vi "PlaceChild.vi"(0 "reference in":refnum<class "VGrid.lvclass">, 5 "error in (no error)":errorcluster) -> (14 "reference out":refnum<class "VGrid.lvclass">, 19 "error out":errorcluster)   [LabVIEW 2019, in "VGrid.lvclass"]
uses:
  VGrid.lvclass
  C:/Users/Taylor.Hillegeist/OneDrive - Ultra/LabVIEW/Pgui2/Pgui_Obj_class/Pgui_Obj.lvclass
  Pgui_Obj_class/Pgui_Obj.lvclass
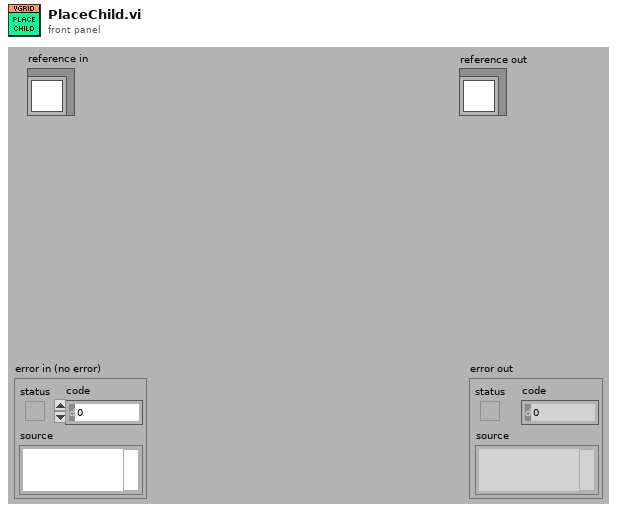
[diagram p1: front panel]
types:
  T1 = cluster{"left":i16, "top":i16, "right":i16, "bottom":i16}
  T2 = typedef "Pgui_Obj.lvclass/ObjectAttributes.ctl" = cluster{"Children":refnum<class "Pgui_Obj.lvclass">[], "Draw Instr":picture, "Params":cluster{"left":i16, "top":i16, "right":i16, "bottom":i16}, "Parent_Pgui_Obj":refnum<class "Pgui_Obj.lvclass">, "MouseOver":bool}
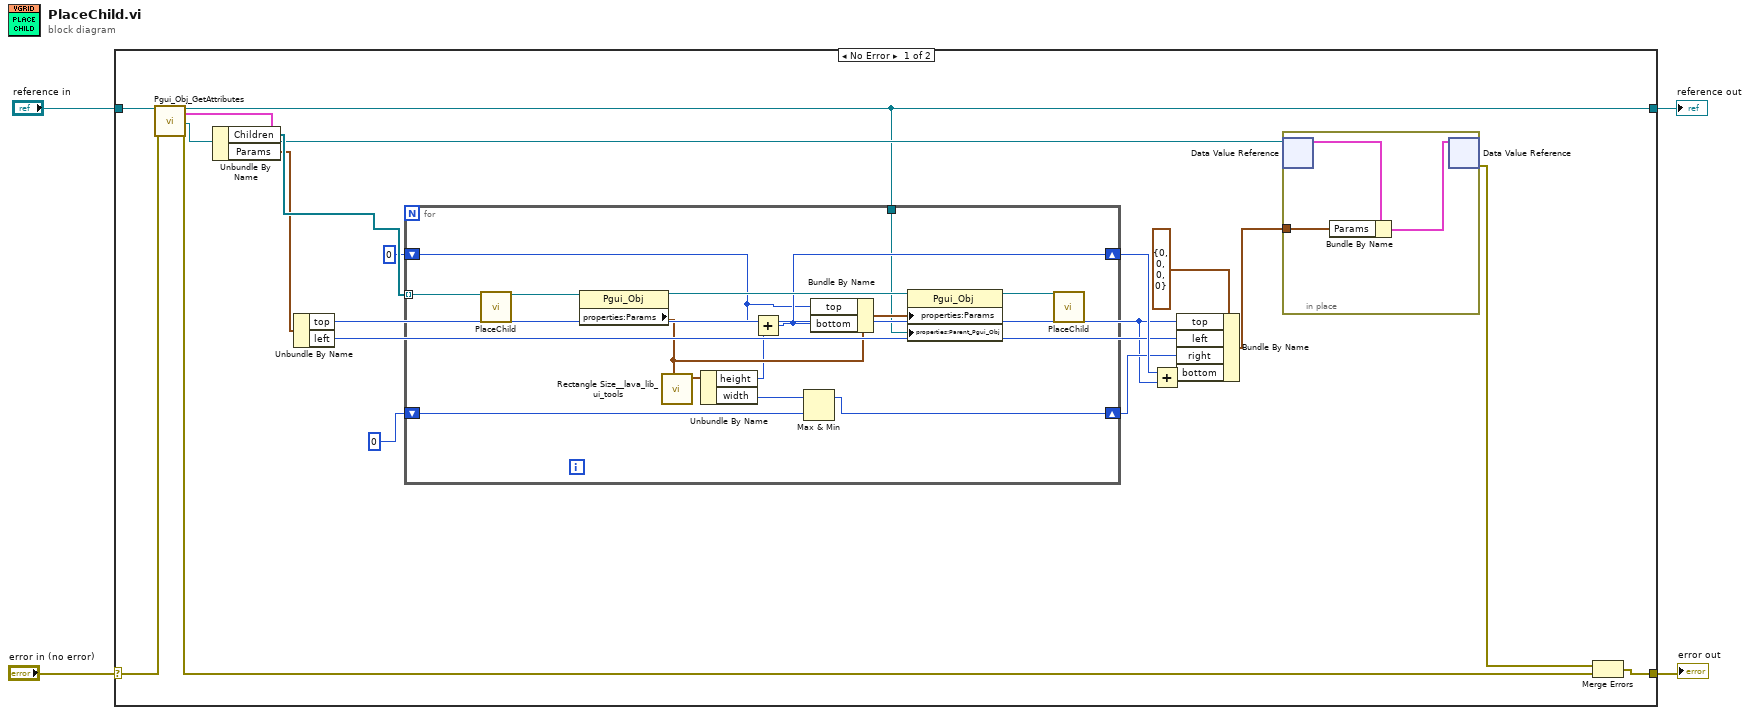
[diagram p0: block diagram]
diagram:
  n1 = case shown="No Error" "error in (no error)" {
    selector: "error in (no error)" -> [w23 w42]
    tunnel: [w20 w42] -> w3
    tunnel: [w8 w41] -> w1
    tunnel: "reference in" -> [w22 w41]
    frame No Error {
      n2 = call "Pgui_Obj_GetAttributes.vi"("reference in"=w22, "error in (no error)"=w23) -> ("reference out"=w8:refnum<class "VGrid.lvclass">, "Data"=w13:T2, "DataRef"=w11:refnum<data-value>, "error out"=w21:errorcluster)  [unwired: 14 in]
      n3 = Unbundle By Name(w13) -> ("Children"=w14:refnum<class "Pgui_Obj.lvclass">[], "Params"=w12:T1)
      n4 = Unbundle By Name(w12) -> ("top"=w5:i16, "left"=w17:i16)
      n5 = for {
        tunnel: w14 -> [w40] mode=indexing
        shift-right: [w37] -> w19
        shift-left: 0 -> [w33]
        shift-right: [w30] -> w18
        shift-left: 0 -> [w32]
        tunnel: w8 -> [w29]
        n6 = call-dynamic "PlaceChild.vi"("reference in"=w40) -> ("reference out"=w28:refnum<class "Pgui_Obj.lvclass">)  [unwired: 17 in, 1 out]
        n7 = property class="Pgui_Obj"(reference=w28) -> (reference out=w39:refnum<class "Pgui_Obj.lvclass">, "properties:Params"=w36:T1)  [unwired: 1 in, 1 out]
        n8 = call <vilib>:"Rectangle Size__lava_lib_ui_tools.vi"("Rectangle"=w36) -> ("Rect Size"=w35:cluster{"width":i32, "height":i32})  [unwired: 8 in, 2 out]
        n9 = Unbundle By Name(w35) -> ("height"=w34:i32, "width"=w31:i32)
        n10 = Add(x=w33, y=w34) -> (x+y=w37:i32)
        n11 = Max & Min(x=w31, y=w32) -> (max(x,y)=w30:i32)  [unwired: 1 out]
        n12 = Bundle By Name(cluster=w36, "top"=w33, "bottom"=w37) -> (w38:T1)
        n13 = property class="Pgui_Obj"(reference=w39, "properties:Params"=w38, "properties:Parent_Pgui_Obj"=w29) -> (reference out=w27:refnum<class "Pgui_Obj.lvclass">)  [unwired: 1 in, 1 out]
        n14 = call-dynamic "PlaceChild.vi"("reference in"=w27) -> ()  [unwired: 17 in, 2 out]
      }
      n15 = Add(x=w19, y=w5) -> (x+y=w6:i32)
      n16 = Bundle By Name(cluster=T1 {"left"=0, "top"=0, "right"=0, "bottom"=0} ("Rectangle"), "top"=w5, "left"=w17, "right"=w18, "bottom"=w6) -> (w10:T1)
      n17 = in-place {
        in-place-border: w10 -> [w24]
        n18 = in-place-dvr #1(w11) -> (w26:T2)  [unwired: 1 out]
        n19 = Bundle By Name(cluster=w26, "Params"=w24) -> (w25:T2)
        n20 = in-place-dvr #1(w25) -> (w9:errorcluster)  [unwired: 1 out]
      }
      n21 = Merge Errors(w9, w21) -> (w20:errorcluster)
    }
    frame Error {
    }
  }
  "error out" <- w3
  "reference out" <- w1
